vi "medicaoIXV.vi"() -> ()   [LabVIEW 2012]
uses:
  <vilib>/Utility/file.llb/Write To Spreadsheet File (string).vi
  <vilib>/Utility/file.llb/Write To Spreadsheet File (DBL).vi
panel:
  out "array":dbl[][](array[numeric])
  in  "Tab Control":enum32{"Entrada de dados", "Saída de dados"}(tab)
  out "ON/OFF":bool
  in  "Pontos":dbl
  in  "Tensão máxima":dbl
  in  "Nome da célula":string
  in  "Local":path
  in  "Delay(ms)":dbl
  in  "Start":bool
  in  "Print Screen":bool
  out "IXV":cluster{"Y":dbl[], "Y":dbl[]}[](graph)
  out "output voltage":dbl
  out "Tensao Atual":dbl
  out "Corrente Atual":dbl
  out "Ponto Atual":i32
  out "TABELA DE DADOS\nTensão(fonte)     Tensão                  Corrente            Pontos":dbl[][](array[numeric]) caption="all rows" format="%0.3f"
  in  "stop":bool
  in  "CorrenteGraph":dbl
  in  "error in (no error)":errorcluster
  out "error out":errorcluster
  in  "TensaoGraph":dbl
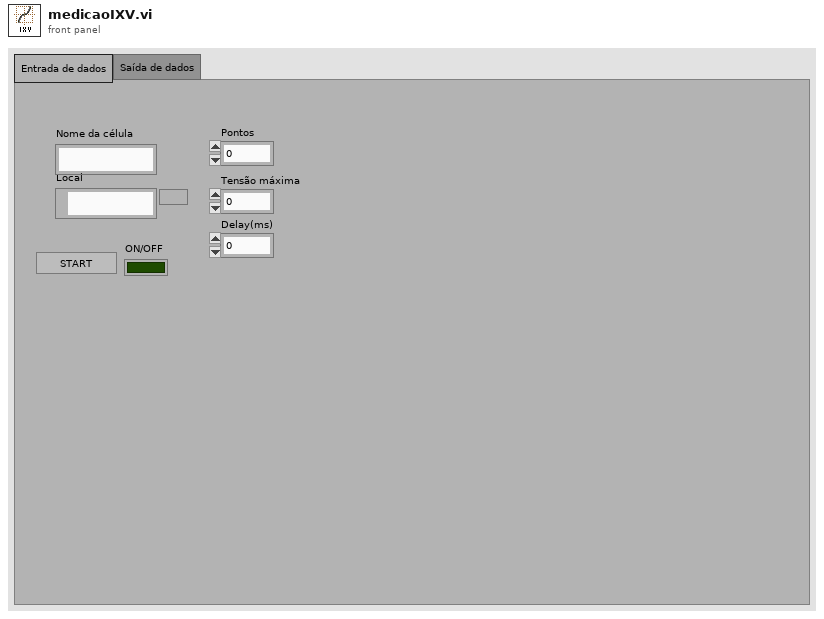
[diagram p1: front panel]
types:
  T1 = typedef "imagedata.ctl" = cluster{"image type":i32, "image depth":i32, "image":u8[], "mask":u8[], "colors":u32[], "Rectangle":cluster{"left":i16, "top":i16, "right":i16, "bottom":i16}}
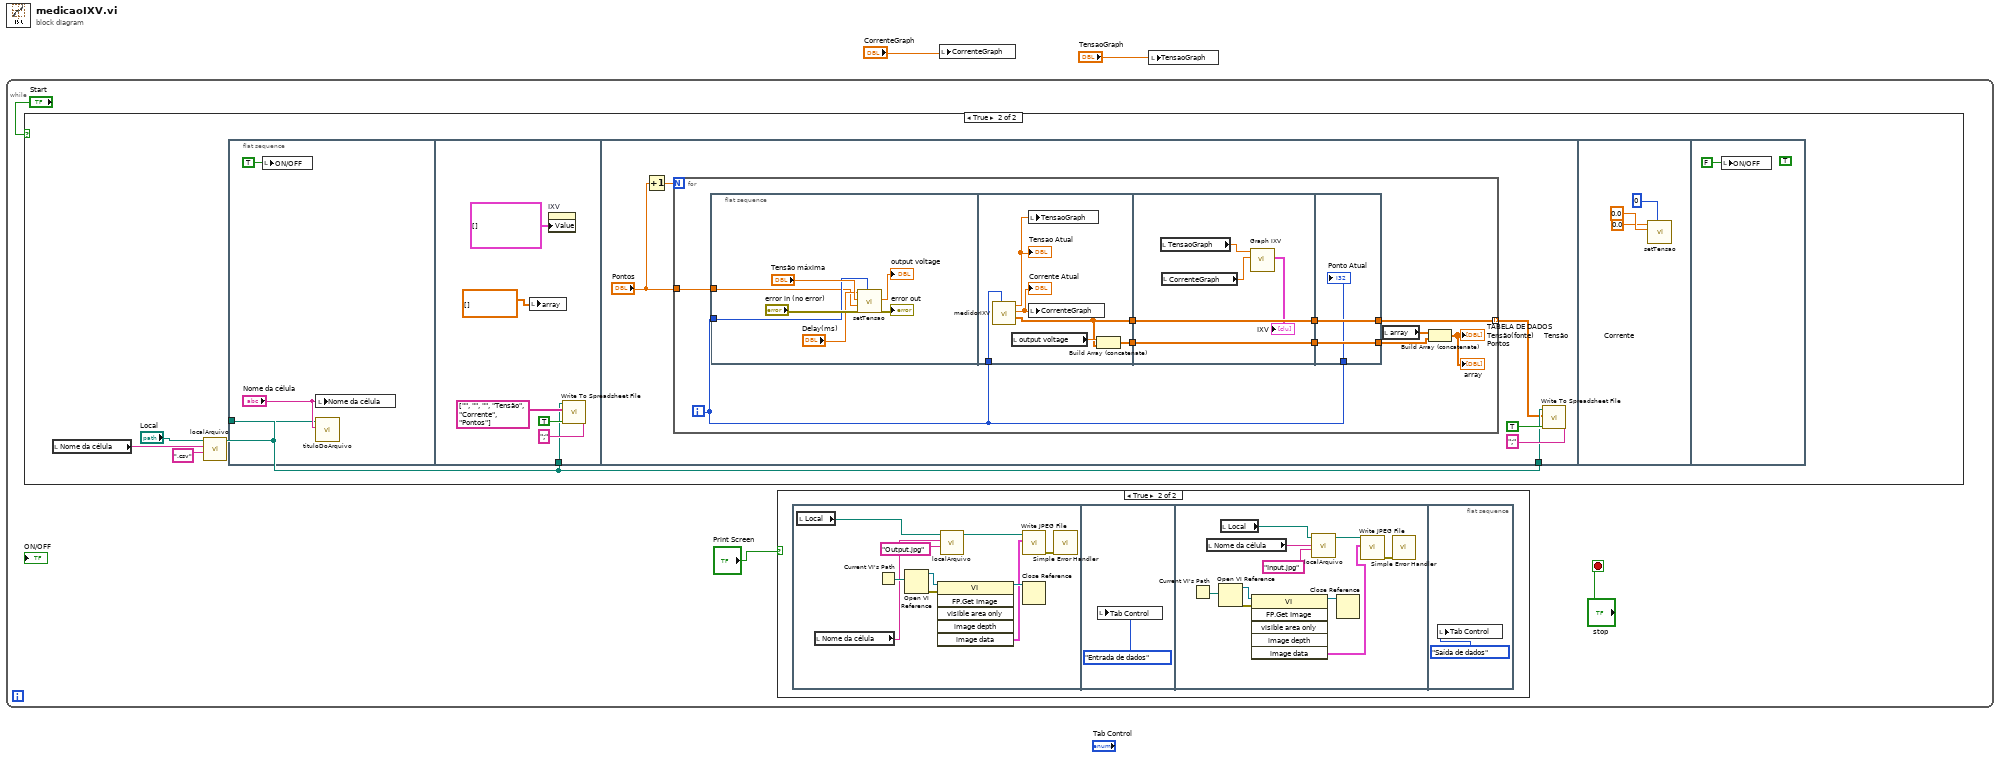
[diagram p0: block diagram]
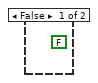
[diagram p3: hidden frame]
diagram:
  n1 = while {
    stop <- "stop" stop-if-true
    n2 = case shown="True" "Start" {
      frame False {
        (unwired) FALSE
      }
      frame True {
        n3 = local read "Nome da célula"() -> (w29:string)
        n4 = call "localArquivo.vi"("extensão"=".csv", "Nome do arquivo"=w29, "Local"="Local") -> ("Path"=w28:path)  [unwired: 8 in]
        n5 = flat-sequence {
          tunnel: w28 -> [w33]
          tunnel: w28 -> [w37]
          tunnel: w28 -> [w44]
          frame #0 {
            n6 = local write "ON/OFF"(TRUE ("ON/OFF")) -> ()
            n7 = local write "Nome da célula"("Nome da célula") -> ()
            n8 = call "tituloDoArquivo.vi"("Nome da célula"="Nome da célula", "file path (dialog if empty)"=w33) -> ()  [unwired: 10 in]
          }
          frame #1 {
            n9 = local write "array"(dbl[][] [] ("array")) -> ()
            n10 = property on="IXV" class="XYGraph (strict)"("Value"=cluster{"Y":dbl[], "Y":dbl[]}[] [] ("IXV")) -> ()  [unwired: 2 in, 2 out]
            n11 = call-poly <vilib>:"Write To Spreadsheet File.vi"("delimiter (\\t)"=";" ("delimiter (\\t)"), "append to file? (new file:F)"=TRUE, "2D data"=string[][] [["", "", ""], ["Tensão", "Corrente", "Pontos"]], "file path (dialog if empty)"=w37) -> ()  [unwired: 4 in, 1 out]
          }
          frame #2 {
            n12 = Increment(x="Pontos") -> (x+1=w43:dbl)
            n13 = for {
              N: w43 -> [_]
              tunnel: [w55] -> w41 mode=indexing
              tunnel: "Pontos" -> [w56]
              i -> [w47]
              n14 = flat-sequence {
                tunnel: w56 -> [w59]
                tunnel: w47 -> [w60]
                tunnel: w47 -> [w69]
                tunnel: [w64] -> w54
                tunnel: [w66] -> w53
                tunnel: w54 -> [w74]
                tunnel: w53 -> [w73]
                tunnel: [w74] -> w49
                tunnel: [w73] -> w48
                tunnel: [w76] -> w52
                tunnel: [w77] -> w55
                tunnel: w49 -> [w77]
                tunnel: w48 -> [w76]
                tunnel: w47 -> [w75]
                frame #0 {
                  n15 = call "setTensao.vi"("Ponto"=w60, "error in (no error)"="error in (no error)", "Pontos"=w59, "Tensão máxima"="Tensão máxima", "delay(ms)"="Delay(ms)") -> ("error out"=→"error out":errorcluster, "output voltage"=→"output voltage":dbl)  [unwired: 5 in]
                }
                frame #1 {
                  n16 = call "medidorIXV.vi"("Ponto"=w69) -> ("Array"=w64:dbl[], "Corrente Atual"=w68:dbl, "Tensao Atual"=w67:dbl)  [unwired: 8 in]
                  "Corrente Atual" <- w68
                  "Tensao Atual" <- w67
                  n17 = local read "output voltage"() -> (w65:dbl)
                  n18 = local write "TensaoGraph"(w67) -> ()
                  n19 = local write "CorrenteGraph"(w68) -> ()
                  n20 = Build Array (concatenate)(w65, w64) -> (w66:dbl[])
                }
                frame #2 {
                  n21 = local read "TensaoGraph"() -> (w72:dbl)
                  n22 = local read "CorrenteGraph"() -> (w71:dbl)
                  n23 = call "Graph IXV"("Y Input"=w71, "X Input"=w72) -> ("XY Graph"=→"IXV":cluster{"Y":dbl[], "Y":dbl[]}[])  [unwired: 3 in, 6 out]
                }
                frame #3 {
                  "Ponto Atual" <- w75
                }
              }
              n24 = local read "array"() -> (w51:dbl[][])
              n25 = Build Array (concatenate)(w51, w52) -> (→"TABELA DE DADOS\nTensão(fonte)     Tensão                  Corrente            Pontos" →"array":dbl[][])
            }
            n26 = call-poly <vilib>:"Write To Spreadsheet File.vi"("delimiter (\\t)"=";" ("delimiter (\\t)"), "append to file? (new file:F)"=TRUE, "2D data"=w41, "file path (dialog if empty)"=w44) -> ()  [unwired: 4 in, 1 out]
          }
          frame #3 {
            n27 = call "setTensao.vi"("Ponto"=0, "Pontos"=0.0, "Tensão máxima"=0.0) -> ()  [unwired: 7 in, 2 out]
          }
          frame #4 {
            (unwired) TRUE
            n28 = local write "ON/OFF"(FALSE) -> ()
          }
        }
      }
    }
    n29 = case shown="True" "Print Screen" {
      frame False {
      }
      frame True {
        n30 = flat-sequence {
          frame #0 {
            n31 = local read "Local"() -> (w7:path)
            n32 = local read "Nome da célula"() -> (w6:string)
            n33 = Current VI's Path() -> (path=w12:path)
            n34 = Open VI Reference(vi path=w12) -> (vi reference=w13:refnum<vi>, error out=w14:errorcluster)  [unwired: 5 in]
            n35 = invoke class="VI" method="FP.Get Image"(reference=w13, error in=w14) -> (reference out=w11:refnum<vi>, "image data"=w10:T1)  [unwired: 4 in, 4 out]
            n36 = call "localArquivo.vi"("extensão"="Output.jpg", "Nome do arquivo"=w6, "Local"=w7) -> ("Path"=w15:path)  [unwired: 8 in]
            n37 = call <vilib>:"Write JPEG File.vi"("image data"=w10, "path to JPEG file"=w15) -> ("error out"=w9:errorcluster)  [unwired: 8 in, 1 out]
            n38 = Close Reference(reference=w11) -> ()  [unwired: 1 in, 1 out]
            n39 = call <vilib>:"Simple Error Handler.vi"("error in (no error)"=w9) -> ()  [unwired: 4 in, 5 out]
          }
          frame #1 {
            n40 = local write "Tab Control"(enum32{"Entrada de dados", "Saída de dados"}."Entrada de dados" ("Tab Control")) -> ()
          }
          frame #2 {
            n41 = Current VI's Path() -> (path=w25:path)
            n42 = local read "Nome da célula"() -> (w18:string)
            n43 = Open VI Reference(vi path=w25) -> (vi reference=w24:refnum<vi>, error out=w23:errorcluster)  [unwired: 5 in]
            n44 = local read "Local"() -> (w17:path)
            n45 = invoke class="VI" method="FP.Get Image"(reference=w24, error in=w23) -> (reference out=w26:refnum<vi>, "image data"=w21:T1)  [unwired: 4 in, 4 out]
            n46 = call "localArquivo.vi"("extensão"="Input.jpg", "Nome do arquivo"=w18, "Local"=w17) -> ("Path"=w20:path)  [unwired: 8 in]
            n47 = Close Reference(reference=w26) -> ()  [unwired: 1 in, 1 out]
            n48 = call <vilib>:"Write JPEG File.vi"("image data"=w21, "path to JPEG file"=w20) -> ("error out"=w22:errorcluster)  [unwired: 8 in, 1 out]
            n49 = call <vilib>:"Simple Error Handler.vi"("error in (no error)"=w22) -> ()  [unwired: 4 in, 5 out]
          }
          frame #3 {
            n50 = local write "Tab Control"(enum32{"Entrada de dados", "Saída de dados"}."Saída de dados" ("Tab Control")) -> ()
          }
        }
      }
    }
  }
  n51 = local write "CorrenteGraph"("CorrenteGraph") -> ()
  n52 = local write "TensaoGraph"("TensaoGraph") -> ()
